vi "GetDevices.vi"() -> (0 "Device Mask":u32 format="%032b")   [LabVIEW 2012]
doc: "This VI can be used to determine the Device Indexes that can be used to utilize ACCES USB devices that are attached to the computer."
uses:
  Windows/System32/AIOUSB.dll
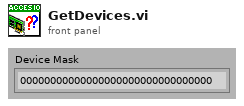
[diagram p1: front panel]
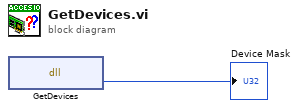
[diagram p0: block diagram]
diagram:
  n1 = dll-call lib="C:/Windows/System32/AIOUSB.dll" fn="GetDevices"() -> (→"Device Mask":u32)  [unwired: 3 in, 2 out]
